vi "Channel Basics Lesson 6.vi"() -> ()   [LabVIEW 2019]
doc: "This VI demonstrates the channel's interaction with Case Structures."
uses:
  <extravilib>/ChannelInstances/Stream-str/Write With Abort.vi
  <extravilib>/ChannelInstances/Stream-str/Read With Abort.vi
  <extravilib>/ChannelInstances/Stream-str/Endpoint.vi
  <extravilib>/ChannelInstances/Stream-str/EndpointRead.vi
  <extravilib>/ChannelInstances/Stream-str/Instantiate.vi
  <extravilib>/ChannelInstances/Stream-str/)Channel.vi
  <resource>/ChannelSupport/_ChannelSupport/WaitIfNeeded.vi
  <extravilib>/ChannelInstances/Stream-str.lvlib
panel:
  out "Sorted Long Strings":string[](array[string])
  out "Sorted Short Strings":string[](array[string])
  in  "Stop":bool
  # "Overview: This VI demonstrates the channel's interaction with Case Structures.\n\nInstructions:\n1. Open the block diagram. Review the lessons presented there.\n2. Run the VI to see that the strings are divided out into separate arrays for short and long strings."
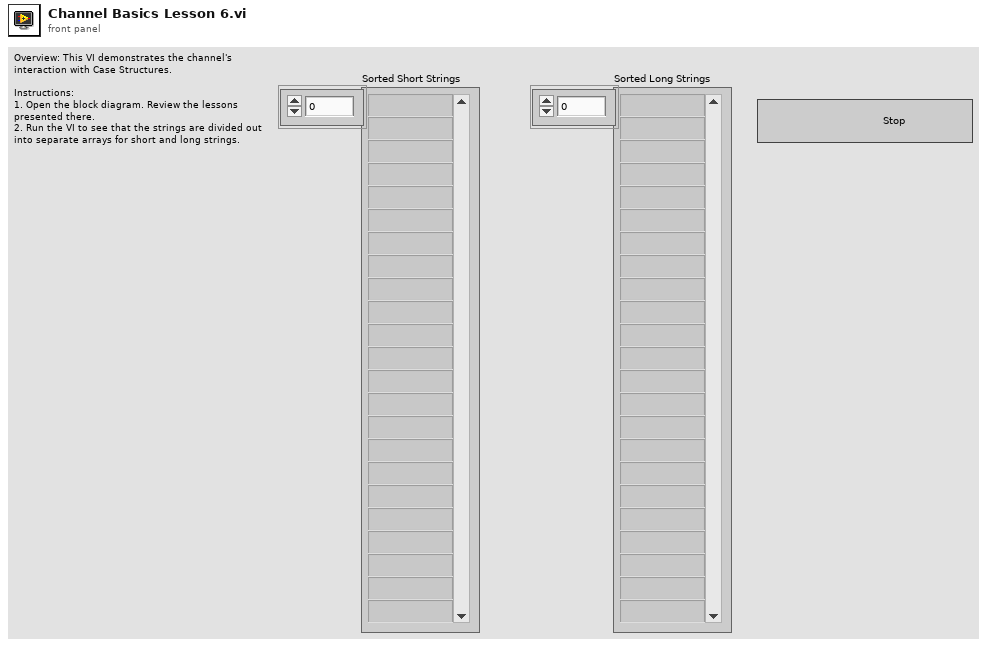
[diagram p1: front panel]
types:
  T1 = typedef "Stream-str.lvlib/)Channel.ctl" = refnum<queue>
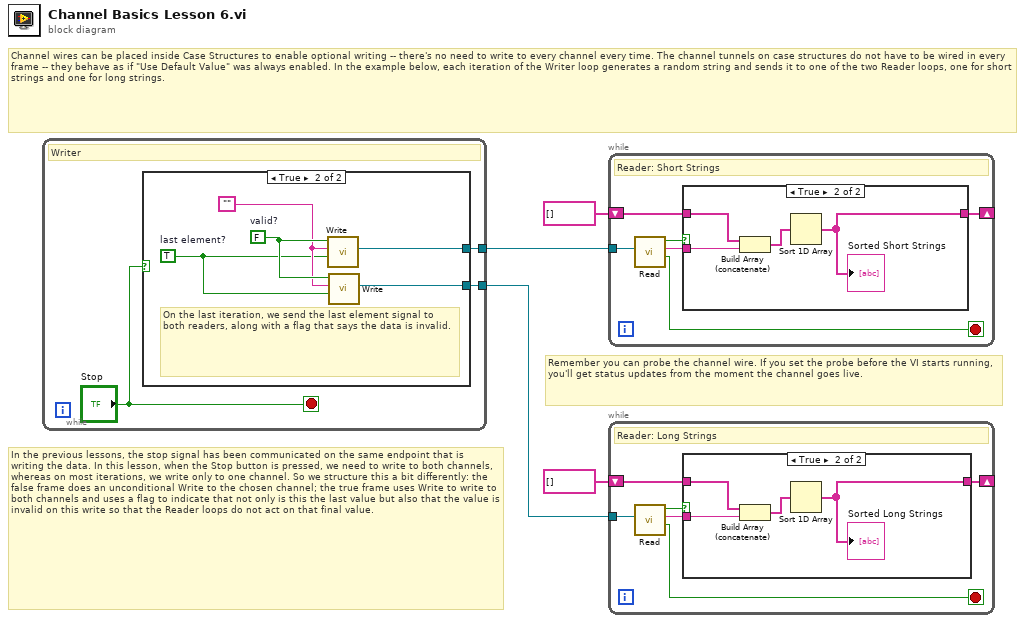
[diagram p0: block diagram]
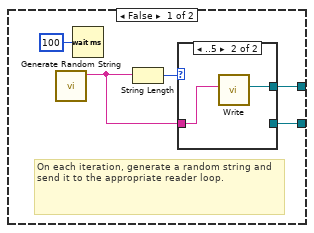
[diagram p2: hidden frame]
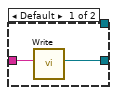
[diagram p3: hidden frame]
diagram:
  # "Remember you can probe the channel wire. If you set the probe before the VI starts running, you'll get status updates from the moment the channel goes live."
  # "In the previous lessons, the stop signal has been communicated on the same endpoint that is  writing the data. In this lesson, when the Stop button is pressed, we need to write to both channels, whereas on most iterations, we write only to one channel. So we structure this a bit differently: the false frame does an unconditional Write to the chosen channel; the true frame uses Write to write to both channels and uses a flag to indicate that not only is this the last value but also that the value is invalid on this write so that the Reader loops do not act on that final value."
  # "Channel wires can be placed inside Case Structures to enable optional writing -- there's no need to write to every channel every time. The channel tunnels on case structures do not have to be wired in every frame -- they behave as if \"Use Default Value\" was always enabled. In the example below, each iteration of the Writer loop generates a random string and sends it to one of the two Reader loops, one for short strings and one for long strings."
  n1 = while {
    tunnel: [w7] -> w1
    tunnel: [w6] -> w4
    stop <- "Stop" stop-if-true
    # "Writer"
    n2 = case shown="True" "Stop" {
      tunnel: [w11 w20] -> w7
      tunnel: [w10 w21] -> w6
      frame False {
        # "On each iteration, generate a random string and send it to the appropriate reader loop."
        n3 = call "Generate Random String.vi"() -> ("Random String"=w8:string)  [unwired: 11 in]
        n4 = Wait (ms)(milliseconds to wait=u32 100) -> ()  [unwired: 1 out]
        n5 = String Length(string=w8) -> (length=w12:i32)
        n6 = case shown="..5" w12 {
          tunnel: w8 -> [w14 w16]
          tunnel: [w13 _] -> w11
          tunnel: [_ w15] -> w10
          frame Default {
            n7 = call <extravilib>:"Write.vi"("element"=w14) -> ("channel"=w13:T1)  [unwired: 8 in, 2 out]
          }
          frame ..5 {
            n8 = call <extravilib>:"Write.vi"("element"=w16) -> ("channel"=w15:T1)  [unwired: 8 in, 2 out]
          }
        }
      }
      frame True {
        w18 = ""
        w19 = FALSE  # valid?
        w17 = TRUE  # last element?
        # "On the last iteration, we send the last element signal to both readers, along with a flag that says the data is invalid."
        n9 = call <extravilib>:"Write.vi"("last element? (F)"=w17, "element"=w18, "element valid? (T)"=w19) -> ("channel"=w21:T1)  [unwired: 6 in, 2 out]
        n10 = call <extravilib>:"Write.vi"("last element? (F)"=w17, "element"=w18, "element valid? (T)"=w19) -> ("channel"=w20:T1)  [unwired: 6 in, 2 out]
      }
    }
  }
  n11 = while {
    tunnel: w4 -> [w22]
    shift-right: [w27] -> _
    shift-left: string[] [] -> [w26]
    stop <- w23 stop-if-true
    # "Reader: Short Strings"
    n12 = call <extravilib>:"Read.vi"("channel"=w22) -> ("last element?"=w23:bool, "element"=w24:string, "element valid?"=w25:bool)  [unwired: 6 in, 2 out]
    n13 = case shown="True" w25 {
      tunnel: [w28 w32] -> w27
      tunnel: w24 -> [_ w30]
      tunnel: w26 -> [w28 w29]
      frame False {
      }
      frame True {
        n14 = Build Array (concatenate)(w29, w30) -> (w31:string[])
        n15 = Sort 1D Array(array=w31) -> (sorted array=w32:string[])
        "Sorted Short Strings" <- w32
      }
    }
  }
  n16 = while {
    tunnel: w1 -> [w36]
    shift-right: [w38] -> _
    shift-left: string[] [] -> [w37]
    stop <- w33 stop-if-true
    # "Reader: Long Strings"
    n17 = call <extravilib>:"Read.vi"("channel"=w36) -> ("last element?"=w33:bool, "element"=w34:string, "element valid?"=w35:bool)  [unwired: 6 in, 2 out]
    n18 = case shown="True" w35 {
      tunnel: [w39 w43] -> w38
      tunnel: w34 -> [_ w41]
      tunnel: w37 -> [w39 w40]
      frame False {
      }
      frame True {
        n19 = Build Array (concatenate)(w40, w41) -> (w42:string[])
        n20 = Sort 1D Array(array=w42) -> (sorted array=w43:string[])
        "Sorted Long Strings" <- w43
      }
    }
  }
